vi "Row_type_selector_string.vi"(1 "Mode":T1) -> (0 "Output string":string)   [LabVIEW 2017]
uses:
  Controls/Multi_run_mode.ctl
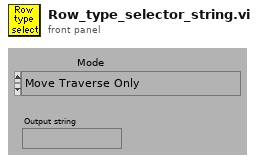
[diagram p1: front panel]
types:
  T1 = typedef "Multi_run_mode.ctl" = enum16{"Move Traverse Only", "Set Tunnel Speed Only", "Set Source Only", "Set Measurement Conditions", "Single Measurement", "Vertical Profile", "Lateral Profile", "Longitudinal Profile", "Explore Volume", "Multi-Axis Profile", "Auto Calibrate", "Meas Fast FID Bkgnd", "Check Beam Power", "Scanning Valve Measurement", "Run VI Named:", "Set ADAM Ch", "Wait (minutes)", "Send Message", "Synchronize With:", "Fall Back to this Row", "Turn Off Row Repeating", "Traverse 3D Volume", "Blank Row", "Jump to Fall Back Row"}
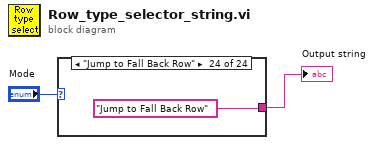
[diagram p0: block diagram]
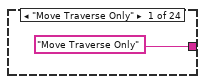
[diagram p2: hidden frame]
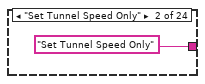
[diagram p3: hidden frame]
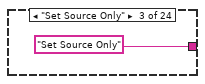
[diagram p4: hidden frame]
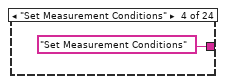
[diagram p5: hidden frame]
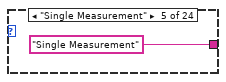
[diagram p6: hidden frame]
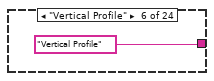
[diagram p7: hidden frame]
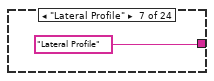
[diagram p8: hidden frame]
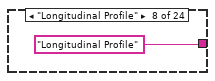
[diagram p9: hidden frame]
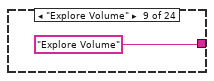
[diagram p10: hidden frame]
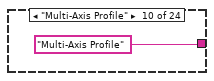
[diagram p11: hidden frame]
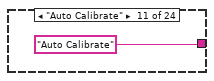
[diagram p12: hidden frame]
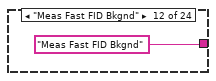
[diagram p13: hidden frame]
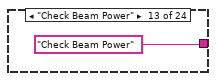
[diagram p14: hidden frame]
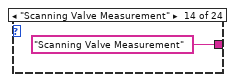
[diagram p15: hidden frame]
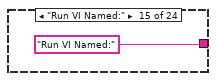
[diagram p16: hidden frame]
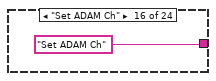
[diagram p17: hidden frame]
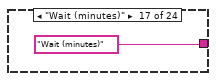
[diagram p18: hidden frame]
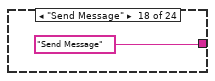
[diagram p19: hidden frame]
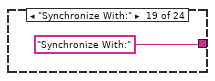
[diagram p20: hidden frame]
diagram:
  n1 = case shown="\"Jump to Fall Back Row\"" "Mode" {
    tunnel: ["Move Traverse Only" "Set Tunnel Speed Only" "Set Source Only" "Set Measurement Conditions" "Single Measurement" "Vertical Profile" "Lateral Profile" "Longitudinal Profile" "Explore Volume" "Multi-Axis Profile" "Auto Calibrate" "Meas Fast FID Bkgnd" "Check Beam Power" "Scanning Valve Measurement" "Run VI Named:" "Set ADAM Ch" "Wait (minutes)" "Send Message" "Synchronize With:" "Fall Back to this Row" "Turn Off Row Repeating" "Traverse 3D Volume" "Blank Row" "Jump to Fall Back Row"] -> w2
    frame "Move Traverse Only" {
    }
    frame "Set Tunnel Speed Only" {
    }
    frame "Set Source Only" {
    }
    frame "Set Measurement Conditions" {
    }
    frame "Single Measurement" {
    }
    frame "Vertical Profile" {
    }
    frame "Lateral Profile" {
    }
    frame "Longitudinal Profile" {
    }
    frame "Explore Volume" {
    }
    frame "Multi-Axis Profile" {
    }
    frame "Auto Calibrate" {
    }
    frame "Meas Fast FID Bkgnd" {
    }
    frame "Check Beam Power" {
    }
    frame "Scanning Valve Measurement" {
    }
    frame "Run VI Named:" {
    }
    frame "Set ADAM Ch" {
    }
    frame "Wait (minutes)" {
    }
    frame "Send Message" {
    }
    frame "Synchronize With:" {
    }
    frame "Fall Back to this Row" {
    }
    frame "Turn Off Row Repeating" {
    }
    frame "Traverse 3D Volume" {
    }
    frame "Blank Row" {
    }
    frame "Jump to Fall Back Row" {
    }
  }
  "Output string" <- w2
